vi "Teleop.vi"(10 "Match Info":T2={"Autonomous Elapsed Seconds"=0.0, "TeleOp Elapsed Seconds"=0.0, "Disabled Elapsed Seconds"=0.0, "Visited Autonomous"=FALSE, "Visited TeleOp"=FALSE, "Visited Disabled"=FALSE, "Autonomous Settings"={"Autonomous Style"=enum."Independent", "VI Refnum"=refnum}}, 11 "Call Context":T3) -> ()   [LabVIEW 2018]
doc: "This VI is called for each TeleOp packet received from the DS where the robot is not disabled. It is often used to read from the joysticks and update I/O or to update setpoints for timed control loops. It should complete and return within 20 milliseconds or it may miss DS packets."
uses:
  <vilib>/Rock Robotics/WPI/DriverStation/WPI_DriverStationDerivedRobotMode.ctl
  <vilib>/Rock Robotics/WPI/DriverStation/WPI_DriverStationMatch Info.ctl
  <vilib>/Rock Robotics/Network Tables/NT Read Boolean.vi
  <vilib>/Rock Robotics/Network Tables/NT Read Number.vi
  <vilib>/Rock Robotics/WPI/Utilities/WPI_GetSetVariantRefNum.vi
  <vilib>/Rock Robotics/Network Tables/NT Write Boolean Array.vi
  <vilib>/Rock Robotics/Network Tables/NT Write Numeric Array.vi
  <vilib>/Rock Robotics/WPI/ThirdParty/Phoenix-LabVIEW/Pigeon IMU/CTRE_PigeonIMU_GetYPR.vi
  <vilib>/Rock Robotics/Network Tables/NT Write Number.vi
  <vilib>/Rock Robotics/WPI/Solenoid/Deprecated/WPI_SolenoidSetBool.vi
  <vilib>/Rock Robotics/WPI/Solenoid/WPI_SolenoidSetEnum.vi
  <vilib>/Rock Robotics/Network Tables/NT Read Numeric Array.vi
  <vilib>/addons/control/pid/pid.llb/PID (DBL).vi
  <vilib>/addons/control/pid/NI_PID_pid.lvlib
panel:
  in  "output range x 2":cluster{"output high":dbl, "output low":dbl}={"output high"=0.5, "output low"=-0.5}
  in  "PID gains x 2":T1={"proportional gain (Kc)"=0.005, "integral time (Ti, min)"=0.0, "derivative time (Td, min)"=0.0}
  in  "output range x":cluster{"output high":dbl, "output low":dbl}={"output high"=0.5, "output low"=-0.5}
  in  "output range z":cluster{"output high":dbl, "output low":dbl}={"output high"=0.75, "output low"=-0.75}
  in  "PID gains x":T1={"proportional gain (Kc)"=0.01, "integral time (Ti, min)"=0.0, "derivative time (Td, min)"=0.0}
  in  "PID gains z":T1={"proportional gain (Kc)"=0.01, "integral time (Ti, min)"=0.0, "derivative time (Td, min)"=0.0}
  out "x":dbl format="%#_13g"
  out "z":dbl format="%#_13g"
  out "Gyro Rotation":dbl
  out "FR  Encoder":dbl
  out "FL Encoder":dbl
  out "BL Encoder":dbl
  out "BR Encoder":dbl
  out "Angle Back Right":dbl
  out "Speed Back Right":dbl
  out "Angle Back Left":dbl
  out "Speed Back Left":dbl
  out "Angle Front Right":dbl
  out "Speed Front Right":dbl
  out "Angle Front Left":dbl
  out "Speed Front Left":dbl
  in  "reverse steer":bool=TRUE
  in  "reverse encoder":bool=TRUE
  in  "ScaleSpeed":dbl=1.0
  in  "upper limit":dbl=0.02
  in  "lower limit":dbl=-0.02
  out "Sample Slider 0":dbl(slide) scale=0.0..5.0
  out "Sample Boolean 1":bool
  out "Sample Boolean 0":bool
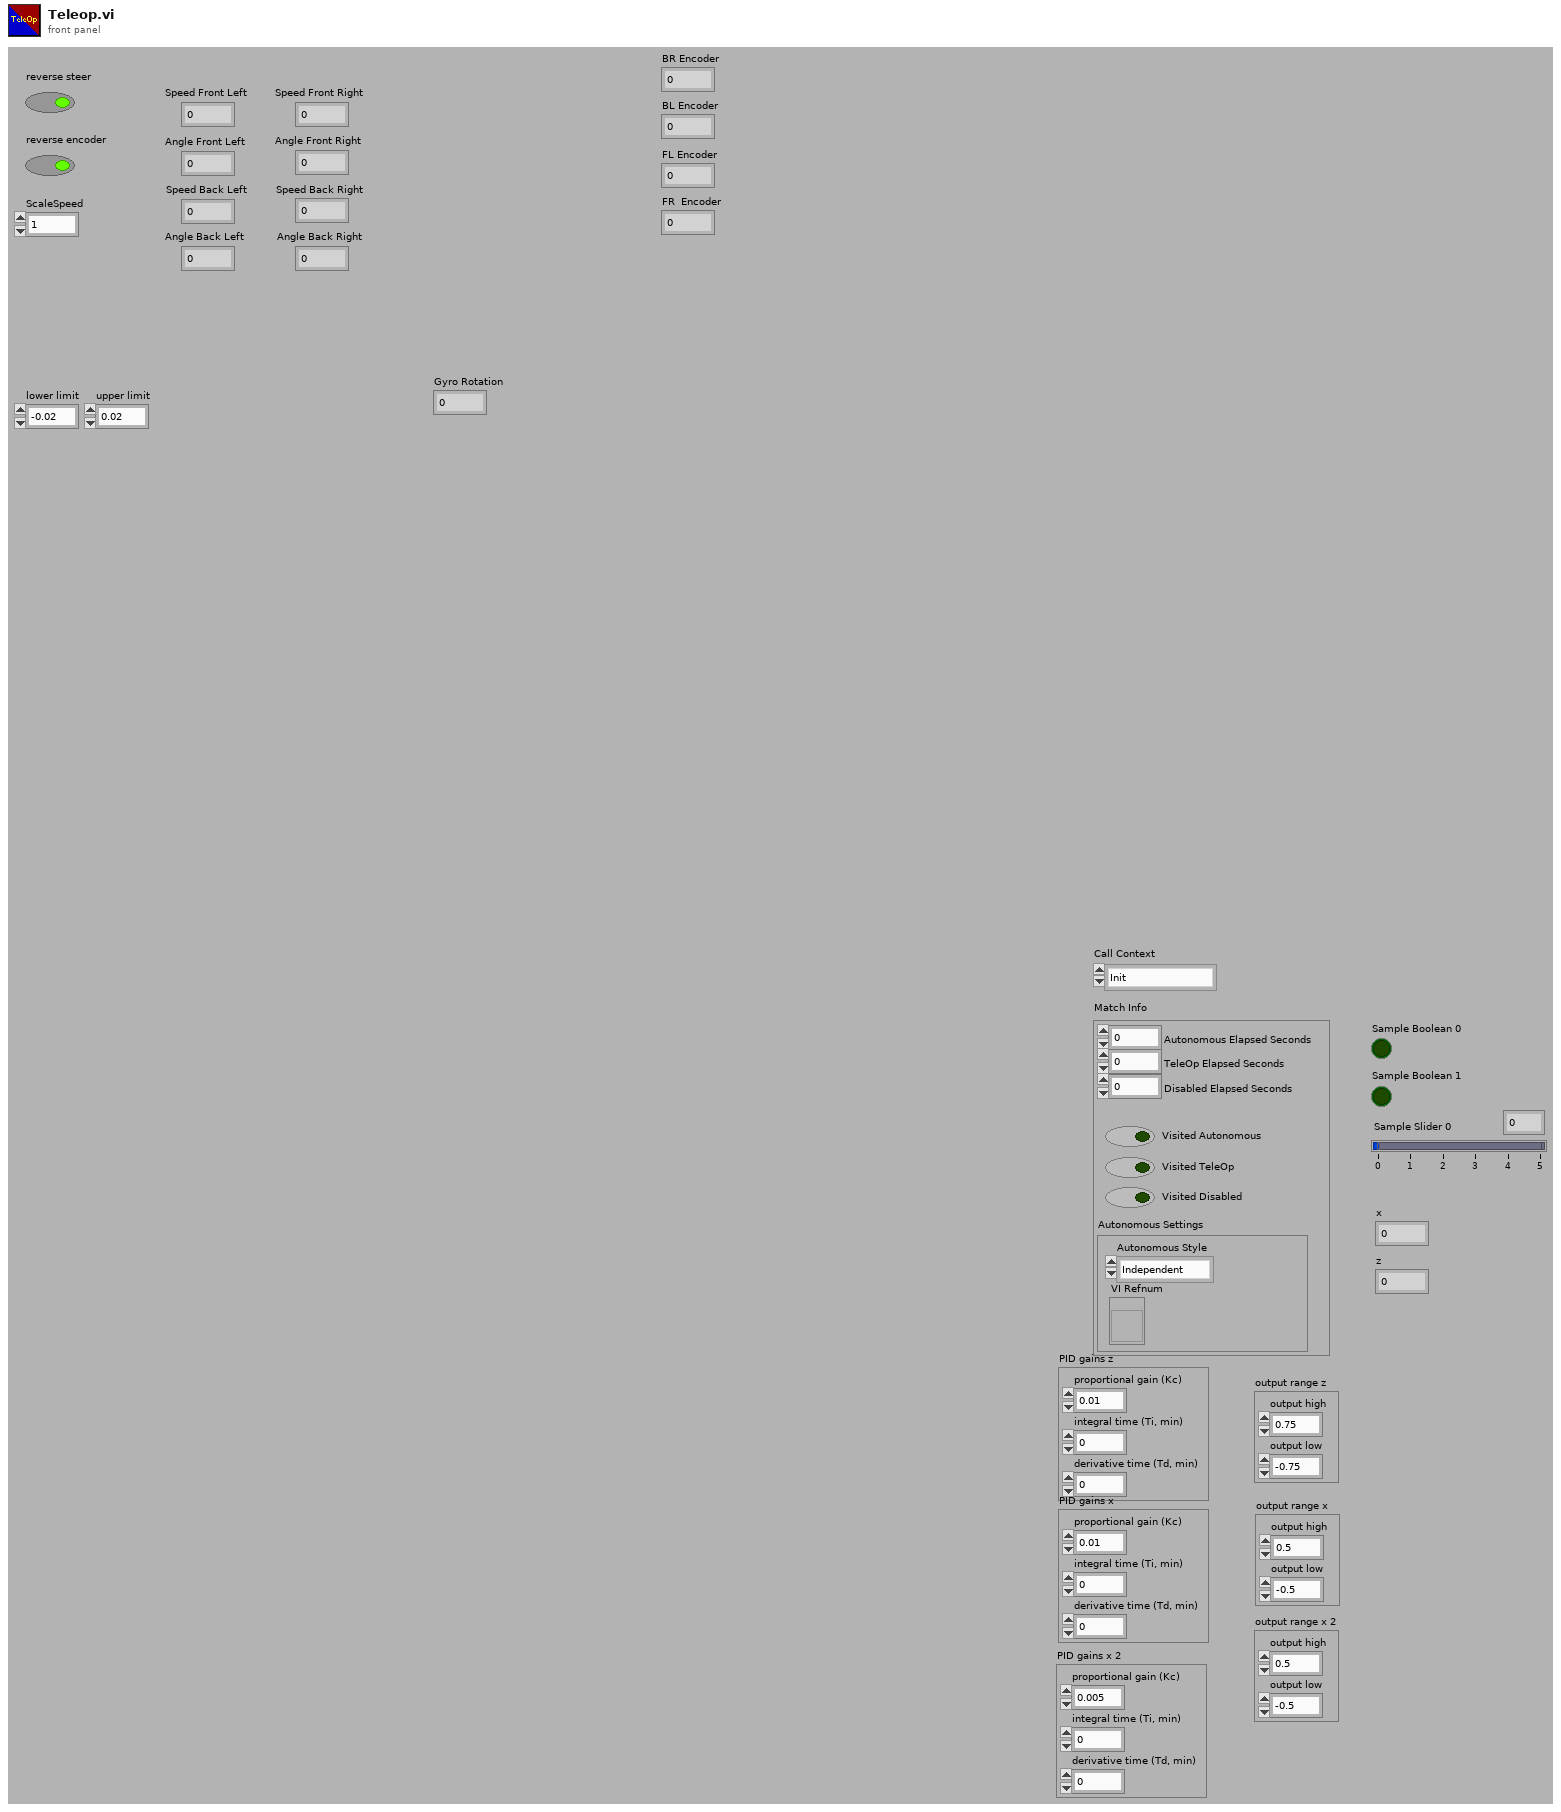
[diagram p1: front panel]
types:
  T1 = cluster{"proportional gain (Kc)":dbl, "integral time (Ti, min)":dbl, "derivative time (Td, min)":dbl}
  T2 = typedef "WPI_DriverStationMatch Info.ctl" = cluster{"Autonomous Elapsed Seconds":dbl, "TeleOp Elapsed Seconds":dbl, "Disabled Elapsed Seconds":dbl, "Visited Autonomous":bool, "Visited TeleOp":bool, "Visited Disabled":bool, "Autonomous Settings":cluster{"Autonomous Style":enum16{"Iterative", "Independent"}, "VI Refnum":refnum<vi>}}
  T3 = typedef "WPI_DriverStationDerivedRobotMode.ctl" = enum16{"Init", "Execute", "Stop"}
  T4 = typedef "WPI_JoystickDevRef.ctl" = cluster{"Device":T5}
  T5 = typedef "WPI_JoystickDeviceEnum.ctl" = enum16{"USB 0", "USB 1", "USB 2", "USB 3", "USB 4", "USB 5"}
  T6 = cluster{"Numeric Array[0]":dbl, "Numeric Array[1]":dbl, "Numeric Array[2]":dbl, "Numeric Array[3]":dbl, "Numeric Array[4]":dbl, "Numeric Array[5]":dbl, "Numeric Array[6]":dbl, "Numeric Array[7]":dbl, "Numeric Array[8]":dbl}
  T7 = typedef "CTRE_PigeonIMU_DeviceRef.ctl" = cluster{"DeviceStatus":errorcluster, "Device Number":u8, "Type":T8, "Device ID":u32, "Handle":u64, "UsageFrame":u32, "Library Path":path}
  T8 = typedef "CTRE_PigeonIMU_ConnectionType.ctl" = u32
  T9 = typedef "WPI_SolenoidDevRef.ctl" = cluster{"DevStatus":errorcluster, "Pneumatics Control Module":u8, "Forward Solenoid Channel":T10, "Reverse Solenoid Channel":T10}
  T10 = typedef "WPI_SolenoidChannel.ctl" = enum8{"Solenoid 0", "Solenoid 1", "Solenoid 2", "Solenoid 3", "Solenoid 4", "Solenoid 5", "Solenoid 6", "Solenoid 7", "Invalid"}
  T11 = typedef "WPI_AnalogChannelDevRef.ctl" = cluster{"DevStatus":errorcluster, "Analog Channel":T12}
  T12 = typedef "FPGA_AIChannel.ctl" = enum8{"AI 0", "AI 1", "AI 2", "AI 3", "AI MXP 0", "AI MXP 1", "AI MXP 2", "AI MXP 3", "Invalid"}
  T13 = typedef "WPI_MotorControlDeviceRef.ctl" = cluster{"DeviceStatus":errorcluster, "Type":T14, "PWM":cluster{"PWM Channel":T15, "DeadBand":T16}, "CAN":cluster{"Device Number":u8, "SetOutput VI Ref":variant, "GetOutput VI Ref":variant, "Enable VI Ref":variant, "Disable VI Ref":variant, "Data":variant}, "Invert":bool, "DIO PWM":cluster{"PWM \"Enable\" Channel":T15, "DIOChannel":T17, "PWM Rate":dbl}}
  T14 = typedef "WPI_MotorControlType.ctl" = enum16{"PWM", "CAN", "DIO PWM"}
  T15 = typedef "FPGA_DIOPWMChannel.ctl" = enum8{"PWM 0", "PWM 1", "PWM 2", "PWM 3", "PWM 4", "PWM 5", "PWM 6", "PWM 7", "PWM 8", "PWM 9", "PWM MXP 0", "PWM MXP 1", "PWM MXP 2", "PWM MXP 3", "PWM MXP 4", "PWM MXP 5", "PWM MXP 6", "PWM MXP 7", "PWM MXP 8", "PWM MXP 9", "Invalid"}
  T16 = typedef "WPI_PWMDeadband.ctl" = cluster{"Name":string, "maxPositivePwm":i32, "minPositivePwm":i32, "centerPwm":i32, "maxNegativePwm":i32, "minNegativePwm":i32, "angularRange":u16}
  T17 = typedef "FPGA_DIOChannel.ctl" = enum8{"DIO 0", "DIO 1", "DIO 2", "DIO 3", "DIO 4", "DIO 5", "DIO 6", "DIO 7", "DIO 8", "DIO 9", "DIO MXP 0", "DIO MXP 1", "DIO MXP 2", "DIO MXP 3", "DIO MXP 4", "DIO MXP 5", "DIO MXP 6", "DIO MXP 7", "DIO MXP 8", "DIO MXP 9", "DIO MXP 10", "DIO MXP 11", "DIO MXP 12", "DIO MXP 13", "DIO MXP 14", "DIO MXP 15", "SPI Port CS1", "SPI Port CS2", "SPI Port CS3", "SPI Port MISO", "SPI Port MOSI", "Invalid"}
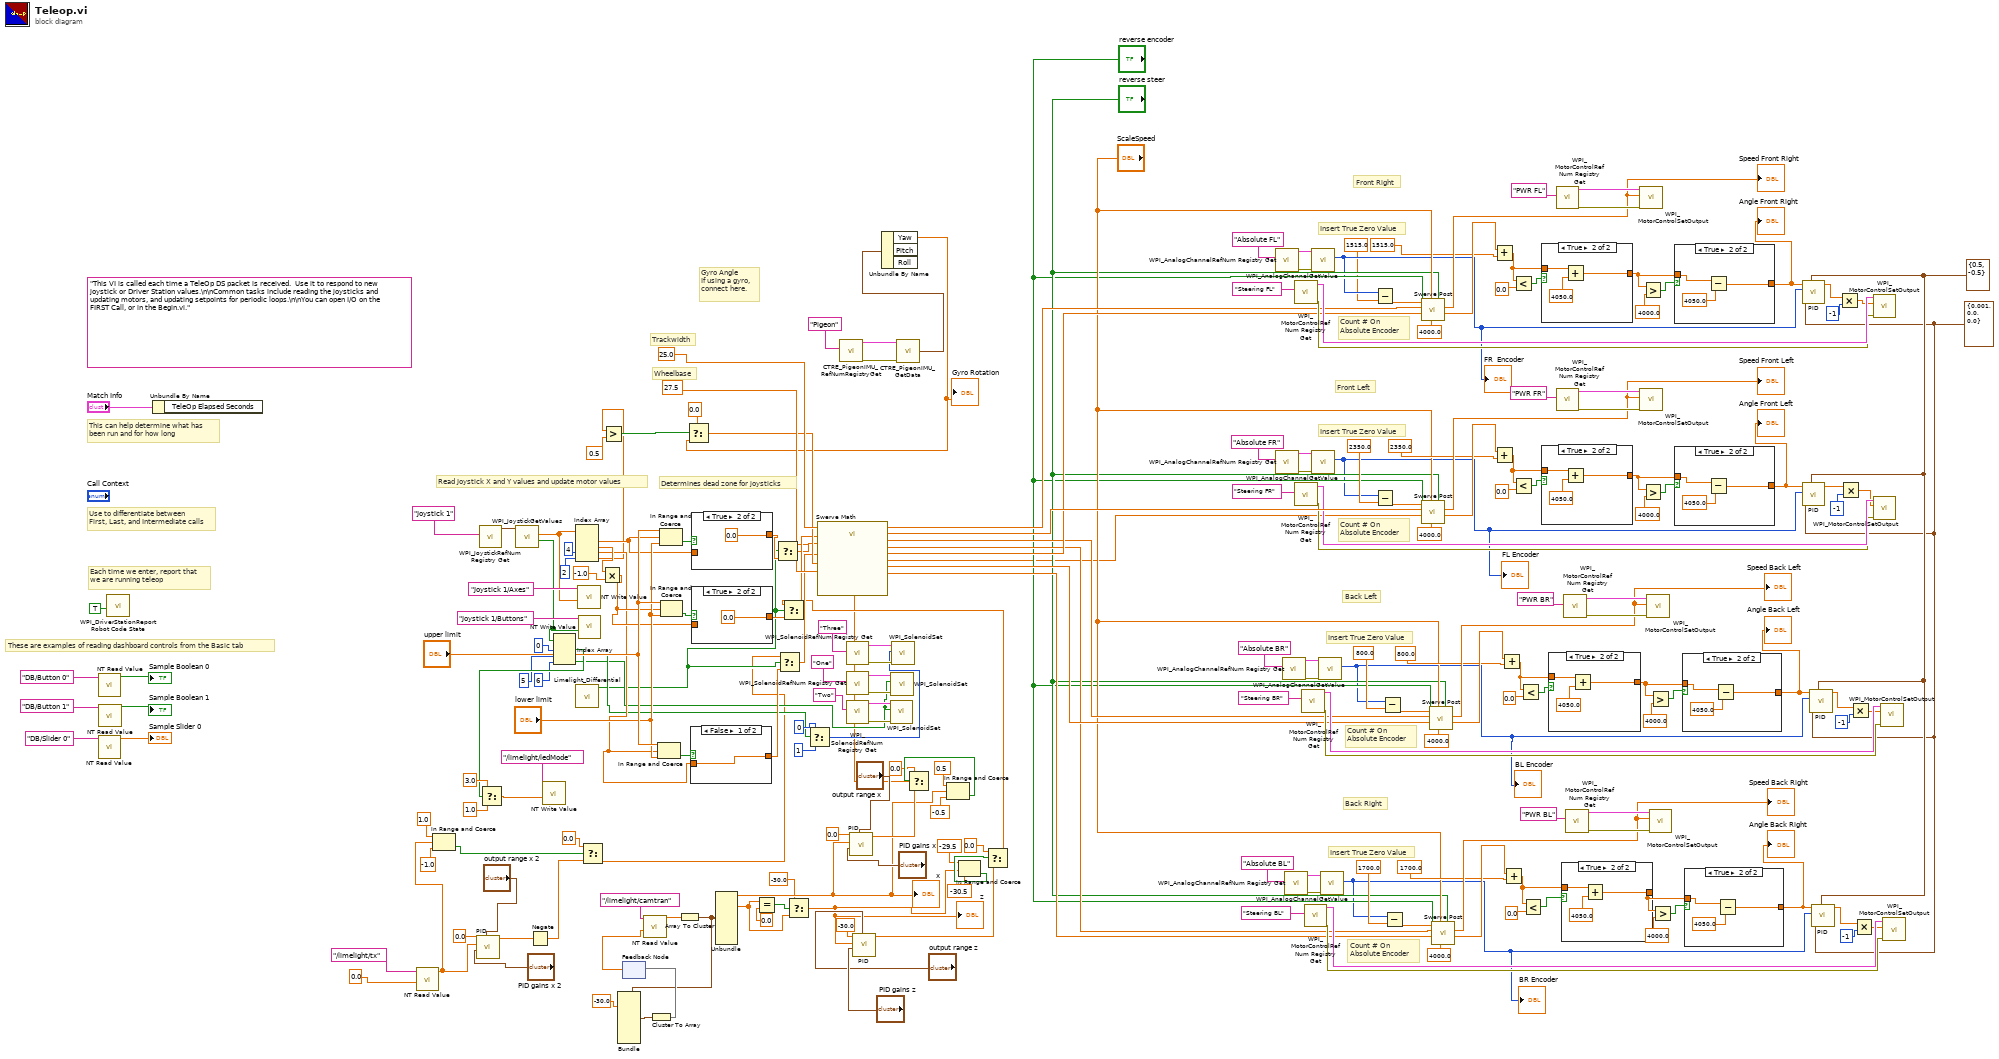
[diagram p0: block diagram]
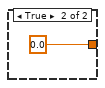
[diagram p10: hidden frame]
diagram:
  w114 = cluster{"output high":dbl, "output low":dbl} {"output high"=0.5, "output low"=-0.5} ("output range 2")
  w113 = T1 {"proportional gain (Kc)"=0.001, "integral time (Ti, min)"=0.0, "derivative time (Td, min)"=0.0} ("PID gains 2")
  (unwired) "This VI is called each time a TeleOp DS packet is received.  Use it to respond to new joystick or Driver Station values.\n\nCommon tasks include reading the joysticks and updating motors, and updating setpoints for periodic loops.\n\nYou can open I/O on the FIRST Call, or in the Begin.vi."
  # "Trackwidth"
  # "Wheelbase"
  # "Count # On \nAbsolute Encoder"
  # "Insert True Zero Value"
  # "Count # On \nAbsolute Encoder"
  # "Insert True Zero Value"
  # "Count # On \nAbsolute Encoder"
  # "Insert True Zero Value"
  # "Count # On \nAbsolute Encoder"
  # "Insert True Zero Value"
  # "Back Right"
  # "Back Left"
  # "Front Left"
  # "Front Right"
  # "Determines dead zone for joysticks"
  # "Gyro Angle\nIf using a gyro,\nconnect here."
  # "Read Joystick X and Y values and update motor values"
  # "These are examples of reading dashboard controls from the Basic tab"
  # "Each time we enter, report that\nwe are running teleop"
  # "Use to differentiate between\nFirst, Last, and Intermediate calls"
  # "This can help determine what has\nbeen run and for how long"
  n1 = call-poly <vilib>:"NT Read Value.vi"("Name"="DB/Button 0" ("refnum name")) -> ("Boolean"=→"Sample Boolean 0":bool)  [unwired: 9 in, 1 out]
  n2 = call-poly <vilib>:"NT Read Value.vi"("Name"="DB/Slider 0" ("refnum name")) -> ("Numeric"=→"Sample Slider 0":dbl)  [unwired: 9 in, 1 out]
  n3 = call-poly <vilib>:"NT Read Value.vi"("Name"="DB/Button 1" ("refnum name")) -> ("Boolean"=→"Sample Boolean 1":bool)  [unwired: 9 in, 1 out]
  n4 = call <vilib>:"WPI_DriverStationReport Robot Code State.vi"("TeleOp"=TRUE ("Autonomous")) -> ()  [unwired: 10 in, 1 out]
  n5 = Unbundle By Name("Match Info") -> ()  [unwired: 1 out]
  n6 = call-poly <vilib>:"NT Read Value.vi"("Default Value"=0.0, "Name"="/limelight/tx") -> ("Numeric"=w25:dbl)  [unwired: 8 in, 1 out]
  n7 = In Range and Coerce(upper limit=1.0, x=w25, lower limit=-1.0) -> (In Range?=w26:bool)  [unwired: 1 out]
  n8 = call-poly <vilib>:"PID.vi"("output range"="output range x 2", "PID gains"="PID gains x 2", "process variable"=w25, "setpoint"=0.0) -> ("output"=w31:dbl)  [unwired: 6 in, 1 out]
  n9 = call <vilib>:"WPI_JoystickRefNum Registry Get.vi"("refnum name"="Joystick 1") -> ("JoystickDevRef"=w219:T4)  [unwired: 1 in, 9 out]
  n10 = call <vilib>:"WPI_JoystickGetValues.vi"("JoystickDevRef"=w219) -> ("Buttons"=w81:bool[], "Axes"=w216:dbl[])  [unwired: 6 in, 3 out]
  n11 = Negate(x=w31) -> (-x=w29:dbl)
  n12 = Index Array(array=w81, index #1=0, index #2=5, index #3=6) -> (element #1=w75:bool, element #2=w51:bool, element #3=w50:bool)
  n13 = Select(t=3.0, s=w75, f=1.0) -> (s? t:f=w78:dbl)
  n14 = call-poly <vilib>:"NT Write Value.vi"("Numeric"=w78, "Name"="/limelight/ledMode") -> ()  [unwired: 9 in, 1 out]
  n15 = Index Array(array=w216, index #3=4, index #4=2) -> (element #1=w89:dbl, element #2=w95:dbl, element #3=w88:dbl, element #4=w84:dbl)  [unwired: 2 in]
  n16 = call "Limelight_Differential.vi"() -> ("TargetValid"=w30:bool)  [unwired: 8 in, 2 out]
  n17 = call-poly <vilib>:"NT Write Value.vi"("Numeric Array"=w216, "Name"="Joystick 1/Axes") -> ()  [unwired: 9 in, 1 out]
  n18 = call-poly <vilib>:"NT Write Value.vi"("Boolean Array"=w81, "Name"="Joystick 1/Buttons") -> ()  [unwired: 9 in, 1 out]
  n19 = Select(t=0.0, s=w26, f=w29) -> (s? t:f=w28:dbl)
  n20 = Multiply(x=w95, y=-1.0) -> (x*y=w94:dbl)
  n21 = Greater?(x=w84, y=0.5) -> (0:w85:bool)
  n22 = feedback #1() -> (w8:dbl[])  [unwired: 1 in]
  n23 = call-poly <vilib>:"NT Read Value.vi"("Default Value"=w8, "Name"="/limelight/camtran") -> ("Numeric Array"=w48:dbl[])  [unwired: 8 in, 1 out]
  n24 = In Range and Coerce(upper limit="upper limit", x=w88, lower limit="lower limit") -> (In Range?=w213:bool)  [unwired: 1 out]
  n25 = In Range and Coerce(upper limit="upper limit", x=w89, lower limit="lower limit") -> (In Range?=w211:bool)  [unwired: 1 out]
  n26 = In Range and Coerce(upper limit="upper limit", x=w94, lower limit="lower limit") -> (In Range?=w212:bool)  [unwired: 1 out]
  n27 = Array To Cluster(array=w48) -> (cluster=w6:T6)
  n28 = Bundle(cluster=w6, "Numeric Array[2]"=-30.0) -> (w10:T6)  [unwired: 8 in]
  n29 = Cluster To Array(cluster=w10) -> (array=w9:dbl[])
  n30 = feedback-in #1(w9) -> ()
  n31 = case shown="False" w213 {
    tunnel: [w229 0.0 ("Gyro Angle")] -> w74
    tunnel: w88 -> [w229 _]
    frame False {
    }
    frame True {
    }
  }
  n32 = case shown="True" w211 {
    tunnel: [w231 0.0 ("Gyro Angle")] -> w41
    tunnel: w89 -> [w231 _]
    frame False {
    }
    frame True {
    }
  }
  n33 = case shown="True" w212 {
    tunnel: [w233 0.0 ("Gyro Angle")] -> w44
    tunnel: w94 -> [w233 _]
    frame False {
    }
    frame True {
    }
  }
  n34 = Unbundle(w6) -> ("Numeric Array[0]"=w14:dbl, "Numeric Array[2]"=w3:dbl)  [unwired: 7 out]
  "x" <- w14
  n35 = Equal?(x=w3, y=0.0) -> (x = y?=w4:bool)
  n36 = Select(t=w28, s=w30, f=w74) -> (s? t:f=w73:dbl)
  n37 = Select(t=-30.0, s=w4, f=w3) -> (s? t:f=w1:dbl)
  "z" <- w1
  n38 = Select(t=0, s=w51, f=1) -> (s? t:f=w52:i32)
  n39 = call <vilib>:"CTRE_PigeonIMU_RefNumRegistryGet.vi"("refnum name"="Pigeon") -> ("error out"=w72:errorcluster, "PigeonIMUDevRef"=w71:T7)  [unwired: 9 in]
  n40 = call <vilib>:"WPI_SolenoidRefNum Registry Get.vi"("refnum name"="Three") -> ("error out"=w61:errorcluster, "SolenoidDevRef"=w60:T9)  [unwired: 9 in]
  n41 = call <vilib>:"WPI_SolenoidRefNum Registry Get.vi"("refnum name"="One") -> ("error out"=w62:errorcluster, "SolenoidDevRef"=w63:T9)  [unwired: 9 in]
  n42 = call <vilib>:"WPI_SolenoidRefNum Registry Get.vi"("refnum name"="Two") -> ("error out"=w65:errorcluster, "SolenoidDevRef"=w64:T9)  [unwired: 9 in]
  n43 = call-poly <vilib>:"PID.vi"("output range"="output range x", "PID gains"="PID gains x", "process variable"=w14, "setpoint"=0.0) -> ("output"=w40:dbl)  [unwired: 6 in, 1 out]
  n44 = call-poly <vilib>:"PID.vi"("output range"="output range z", "PID gains"="PID gains z", "process variable"=w1, "setpoint"=-30.0) -> ("output"=w43:dbl)  [unwired: 6 in, 1 out]
  n45 = call-poly <vilib>:"WPI_SolenoidSet.vi"("error in (no error)"=w65, "Value"=w50, "SolenoidDevRef"=w64) -> ()  [unwired: 7 in, 2 out]
  n46 = call-poly <vilib>:"WPI_SolenoidSet.vi"("error in (no error)"=w62, "Value"=w50, "SolenoidDevRef"=w63) -> ()  [unwired: 7 in, 2 out]
  n47 = call-poly <vilib>:"WPI_SolenoidSet.vi"("error in (no error)"=w61, "Value"=w52, "SolenoidDevRef"=w60) -> ()  [unwired: 7 in, 2 out]
  n48 = call-poly <vilib>:"CTRE_PigeonIMU_GetData.vi"("error in (no error)"=w72, "PigeonIMUDevRef"=w71) -> ("Yaw Pitch Roll"=w70:cluster{"Yaw":dbl, "Pitch":dbl, "Roll":dbl})  [unwired: 7 in, 2 out]
  n49 = Unbundle By Name(w70) -> ("Yaw"=w68:dbl)  [unwired: 2 out]
  "Gyro Rotation" <- w68
  n50 = Select(t=0.0 ("Gyro Angle"), s=w85, f=w68) -> (s? t:f=w83:dbl)
  n51 = In Range and Coerce(upper limit=0.5, x=w14, lower limit=-0.5) -> (In Range?=w13:bool)  [unwired: 1 out]
  n52 = Select(t=0.0, s=w13, f=w40) -> (s? t:f=w17:dbl)
  n53 = Select(t=w17, s=w30, f=w41) -> (s? t:f=w42:dbl)
  n54 = In Range and Coerce(upper limit=-29.5, x=w1, lower limit=-30.5) -> (In Range?=w20:bool)  [unwired: 1 out]
  n55 = Select(t=0.0, s=w20, f=w43) -> (s? t:f=w22:dbl)
  n56 = Select(t=w22, s=w30, f=w44) -> (s? t:f=w45:dbl)
  n57 = call "Swerve Math.vi"("Trackwidth (W)"=25.0, "Wheelbase (L)"=27.5, "Y -FWD"=w45, "X1 STR"=w42, "X2 RCW"=w73, "Gyro Angle in degrees"=w83) -> ("wa3"=w146:dbl, "wa4"=w121:dbl, "ws1"=w168:dbl, "ws2"=w208:dbl, "ws3"=w145:dbl, "ws4"=w122:dbl, "wa2"=w96:dbl, "wa1"=w169:dbl)  [unwired: 2 in]
  n58 = call <vilib>:"WPI_AnalogChannelRefNum Registry Get.vi"("refnum name"="Absolute FL") -> ("error out"=w183:errorcluster, "AIDeviceRef"=w182:T11)  [unwired: 9 in]
  n59 = call <vilib>:"WPI_AnalogChannelRefNum Registry Get.vi"("refnum name"="Absolute FR") -> ("error out"=w204:errorcluster, "AIDeviceRef"=w203:T11)  [unwired: 9 in]
  n60 = call <vilib>:"WPI_AnalogChannelRefNum Registry Get.vi"("refnum name"="Absolute BR") -> ("error out"=w162:errorcluster, "AIDeviceRef"=w161:T11)  [unwired: 9 in]
  n61 = call <vilib>:"WPI_AnalogChannelRefNum Registry Get.vi"("refnum name"="Absolute BL") -> ("error out"=w139:errorcluster, "AIDeviceRef"=w138:T11)  [unwired: 9 in]
  n62 = call <vilib>:"WPI_MotorControlRefNum Registry Get.vi"("refnum name"="Steering FL") -> ("error out"=w177:errorcluster, "MotorControlDevRef"=w178:T13)  [unwired: 9 in]
  n63 = call <vilib>:"WPI_MotorControlRefNum Registry Get.vi"("refnum name"="Steering FR") -> ("error out"=w196:errorcluster, "MotorControlDevRef"=w197:T13)  [unwired: 9 in]
  n64 = call <vilib>:"WPI_MotorControlRefNum Registry Get.vi"("refnum name"="Steering BR") -> ("error out"=w154:errorcluster, "MotorControlDevRef"=w155:T13)  [unwired: 9 in]
  n65 = call <vilib>:"WPI_MotorControlRefNum Registry Get.vi"("refnum name"="Steering BL") -> ("error out"=w131:errorcluster, "MotorControlDevRef"=w132:T13)  [unwired: 9 in]
  n66 = call <vilib>:"WPI_AnalogChannelGetValue.vi"("error in (no error)"=w183, "AIDeviceRef"=w182) -> ("Value"=w115:i16)  [unwired: 7 in, 2 out]
  "FR  Encoder" <- w115
  n67 = call <vilib>:"WPI_AnalogChannelGetValue.vi"("error in (no error)"=w204, "AIDeviceRef"=w203) -> ("Value"=w116:i16)  [unwired: 7 in, 2 out]
  "FL Encoder" <- w116
  n68 = call <vilib>:"WPI_AnalogChannelGetValue.vi"("error in (no error)"=w162, "AIDeviceRef"=w161) -> ("Value"=w117:i16)  [unwired: 7 in, 2 out]
  "BL Encoder" <- w117
  n69 = call <vilib>:"WPI_AnalogChannelGetValue.vi"("error in (no error)"=w139, "AIDeviceRef"=w138) -> ("Value"=w118:i16)  [unwired: 7 in, 2 out]
  "BR Encoder" <- w118
  n70 = Subtract(x=w115, y=1515.0) -> (x-y=w180:dbl)
  n71 = Subtract(x=w116, y=2350.0) -> (x-y=w200:dbl)
  n72 = Subtract(x=w117, y=800.0) -> (x-y=w158:dbl)
  n73 = Subtract(x=w118, y=1700.0) -> (x-y=w135:dbl)
  n74 = call "Swerve Post.vi"("reverse encoder"="reverse encoder", "reverse steer"="reverse steer", "gear ratio"=4000.0, "ScaleSpeed"="ScaleSpeed", "wa in"=w169, "ws in"=w168, "encoder in"=w180) -> ("wa out"=w179:dbl, "ws out 0-1"=w184:dbl)  [unwired: 3 in]
  "Speed Front Right" <- w184
  n75 = call "Swerve Post.vi"("reverse encoder"="reverse encoder", "reverse steer"="reverse steer", "gear ratio"=4000.0, "ScaleSpeed"="ScaleSpeed", "wa in"=w96, "ws in"=w208, "encoder in"=w200) -> ("wa out"=w199:dbl, "ws out 0-1"=w205:dbl)  [unwired: 3 in]
  "Speed Front Left" <- w205
  n76 = call "Swerve Post.vi"("reverse encoder"="reverse encoder", "reverse steer"="reverse steer", "gear ratio"=4000.0, "ScaleSpeed"="ScaleSpeed", "wa in"=w146, "ws in"=w145, "encoder in"=w158) -> ("wa out"=w157:dbl, "ws out 0-1"=w163:dbl)  [unwired: 3 in]
  "Speed Back Left" <- w163
  n77 = call "Swerve Post.vi"("reverse encoder"="reverse encoder", "reverse steer"="reverse steer", "gear ratio"=4000.0, "ScaleSpeed"="ScaleSpeed", "wa in"=w121, "ws in"=w122, "encoder in"=w135) -> ("wa out"=w134:dbl, "ws out 0-1"=w140:dbl)  [unwired: 3 in]
  "Speed Back Right" <- w140
  n78 = Add(x=w179, y=1515.0) -> (x+y=w174:dbl)
  n79 = Add(x=w199, y=2350.0) -> (x+y=w193:dbl)
  n80 = Add(x=w157, y=800.0) -> (x+y=w151:dbl)
  n81 = Add(x=w134, y=1700.0) -> (x+y=w128:dbl)
  n82 = Less?(x=w174, y=0.0) -> (x < y?=w176:bool)
  n83 = Less?(x=w193, y=0.0) -> (x < y?=w195:bool)
  n84 = Less?(x=w151, y=0.0) -> (x < y?=w153:bool)
  n85 = Less?(x=w128, y=0.0) -> (x < y?=w130:bool)
  n86 = case shown="True" w176 {
    tunnel: w174 -> [w235 w238]
    tunnel: [w235 w236] -> w171
    frame False {
    }
    frame True {
      n87 = Add(x=w238, y=4050.0) -> (x+y=w236:dbl)
    }
  }
  n88 = case shown="True" w195 {
    tunnel: w193 -> [w239 w242]
    tunnel: [w239 w240] -> w190
    frame False {
    }
    frame True {
      n89 = Add(x=w242, y=4050.0) -> (x+y=w240:dbl)
    }
  }
  n90 = case shown="True" w153 {
    tunnel: w151 -> [w243 w246]
    tunnel: [w243 w244] -> w148
    frame False {
    }
    frame True {
      n91 = Add(x=w246, y=4050.0) -> (x+y=w244:dbl)
    }
  }
  n92 = call <vilib>:"WPI_MotorControlRefNum Registry Get.vi"("refnum name"="PWR FL") -> ("error out"=w185:errorcluster, "MotorControlDevRef"=w186:T13)  [unwired: 9 in]
  n93 = call <vilib>:"WPI_MotorControlRefNum Registry Get.vi"("refnum name"="PWR FR") -> ("error out"=w206:errorcluster, "MotorControlDevRef"=w207:T13)  [unwired: 9 in]
  n94 = case shown="True" w130 {
    tunnel: w128 -> [w247 w250]
    tunnel: [w247 w248] -> w125
    frame False {
    }
    frame True {
      n95 = Add(x=w250, y=4050.0) -> (x+y=w248:dbl)
    }
  }
  n96 = call <vilib>:"WPI_MotorControlRefNum Registry Get.vi"("refnum name"="PWR BR") -> ("error out"=w164:errorcluster, "MotorControlDevRef"=w165:T13)  [unwired: 9 in]
  n97 = call <vilib>:"WPI_MotorControlRefNum Registry Get.vi"("refnum name"="PWR BL") -> ("error out"=w141:errorcluster, "MotorControlDevRef"=w142:T13)  [unwired: 9 in]
  n98 = call <vilib>:"WPI_MotorControlSetOutput.vi"("error in (no error)"=w185, "Output"=w184, "MotorControlDevRef"=w186) -> ()  [unwired: 6 in, 3 out]
  n99 = call <vilib>:"WPI_MotorControlSetOutput.vi"("error in (no error)"=w206, "Output"=w205, "MotorControlDevRef"=w207) -> ()  [unwired: 6 in, 3 out]
  n100 = Greater?(x=w171, y=4000.0) -> (0:w173:bool)
  n101 = Greater?(x=w190, y=4000.0) -> (0:w192:bool)
  n102 = call <vilib>:"WPI_MotorControlSetOutput.vi"("error in (no error)"=w164, "Output"=w163, "MotorControlDevRef"=w165) -> ()  [unwired: 6 in, 3 out]
  n103 = Greater?(x=w148, y=4000.0) -> (0:w150:bool)
  n104 = call <vilib>:"WPI_MotorControlSetOutput.vi"("error in (no error)"=w141, "Output"=w140, "MotorControlDevRef"=w142) -> ()  [unwired: 6 in, 3 out]
  n105 = Greater?(x=w125, y=4000.0) -> (0:w127:bool)
  n106 = case shown="True" w173 {
    tunnel: w171 -> [w251 w254]
    tunnel: [w251 w252] -> w109
    frame False {
    }
    frame True {
      n107 = Subtract(x=w254, y=4050.0) -> (x-y=w252:dbl)
    }
  }
  "Angle Front Right" <- w109
  n108 = case shown="True" w192 {
    tunnel: w190 -> [w255 w258]
    tunnel: [w255 w256] -> w110
    frame False {
    }
    frame True {
      n109 = Subtract(x=w258, y=4050.0) -> (x-y=w256:dbl)
    }
  }
  "Angle Front Left" <- w110
  n110 = case shown="True" w150 {
    tunnel: w148 -> [w259 w262]
    tunnel: [w259 w260] -> w111
    frame False {
    }
    frame True {
      n111 = Subtract(x=w262, y=4050.0) -> (x-y=w260:dbl)
    }
  }
  "Angle Back Left" <- w111
  n112 = case shown="True" w127 {
    tunnel: w125 -> [w263 w266]
    tunnel: [w263 w264] -> w112
    frame False {
    }
    frame True {
      n113 = Subtract(x=w266, y=4050.0) -> (x-y=w264:dbl)
    }
  }
  "Angle Back Right" <- w112
  n114 = call-poly <vilib>:"PID.vi"("output range"=w114, "PID gains"=w113, "process variable"=w115, "setpoint"=w109) -> ("output"=w98:dbl)  [unwired: 6 in, 1 out]
  n115 = call-poly <vilib>:"PID.vi"("output range"=w114, "PID gains"=w113, "process variable"=w116, "setpoint"=w110) -> ("output"=w108:dbl)  [unwired: 6 in, 1 out]
  n116 = call-poly <vilib>:"PID.vi"("output range"=w114, "PID gains"=w113, "process variable"=w117, "setpoint"=w111) -> ("output"=w101:dbl)  [unwired: 6 in, 1 out]
  n117 = call-poly <vilib>:"PID.vi"("output range"=w114, "PID gains"=w113, "process variable"=w118, "setpoint"=w112) -> ("output"=w104:dbl)  [unwired: 6 in, 1 out]
  n118 = Multiply(x=w98, y=-1) -> (x*y=w99:dbl)
  n119 = Multiply(x=w108, y=-1) -> (x*y=w107:dbl)
  n120 = Multiply(x=w101, y=-1) -> (x*y=w102:dbl)
  n121 = Multiply(x=w104, y=-1) -> (x*y=w105:dbl)
  n122 = call <vilib>:"WPI_MotorControlSetOutput.vi"("error in (no error)"=w177, "Output"=w99, "MotorControlDevRef"=w178) -> ()  [unwired: 6 in, 3 out]
  n123 = call <vilib>:"WPI_MotorControlSetOutput.vi"("error in (no error)"=w196, "Output"=w107, "MotorControlDevRef"=w197) -> ()  [unwired: 6 in, 3 out]
  n124 = call <vilib>:"WPI_MotorControlSetOutput.vi"("error in (no error)"=w154, "Output"=w102, "MotorControlDevRef"=w155) -> ()  [unwired: 6 in, 3 out]
  n125 = call <vilib>:"WPI_MotorControlSetOutput.vi"("error in (no error)"=w131, "Output"=w105, "MotorControlDevRef"=w132) -> ()  [unwired: 6 in, 3 out]
